vi "111_Setting.vi"() -> ()   [LabVIEW 2018]
panel:
  in  "偏移设定":T1
  in  "压销力":sgl[](array[numeric])
  in  "压销位移":sgl[](array[numeric])
  in  "内泄露":sgl[](array[numeric])
  in  "输入轴扭矩传感器":sgl[](array[numeric])
  in  "油压值":sgl[](array[numeric])
  # "传感器配置"
  # "量程下限"
  # "量程下限"
  # "量程下限"
  # "量程上限"
  # "量程上限"
  # "量程上限"
  # "量程下限"
  # "量程下限"
  # "量程上限"
  # "量程上限"
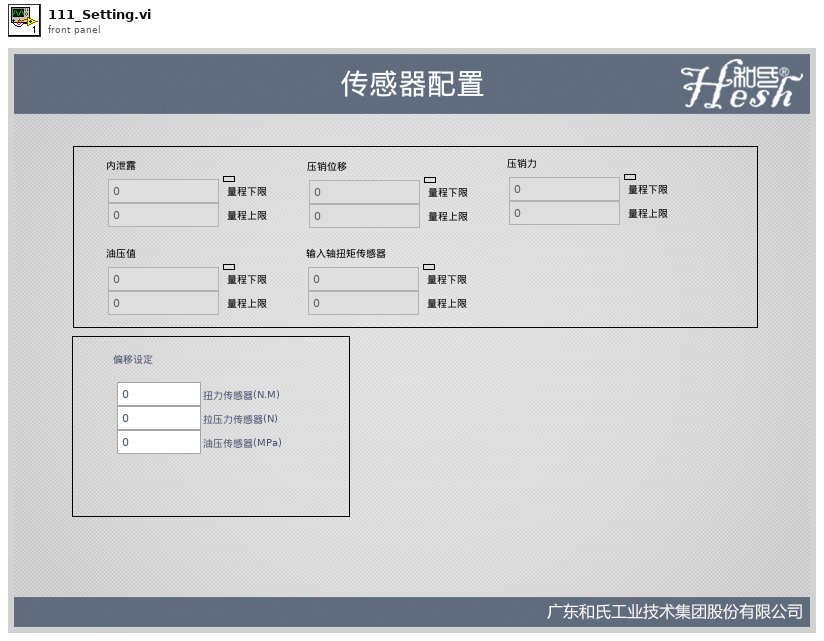
[diagram p1: front panel]
types:
  T1 = cluster{"扭力传感器(N.M)":dbl, "拉压力传感器(N)":dbl, "油压传感器(MPa) ":dbl}
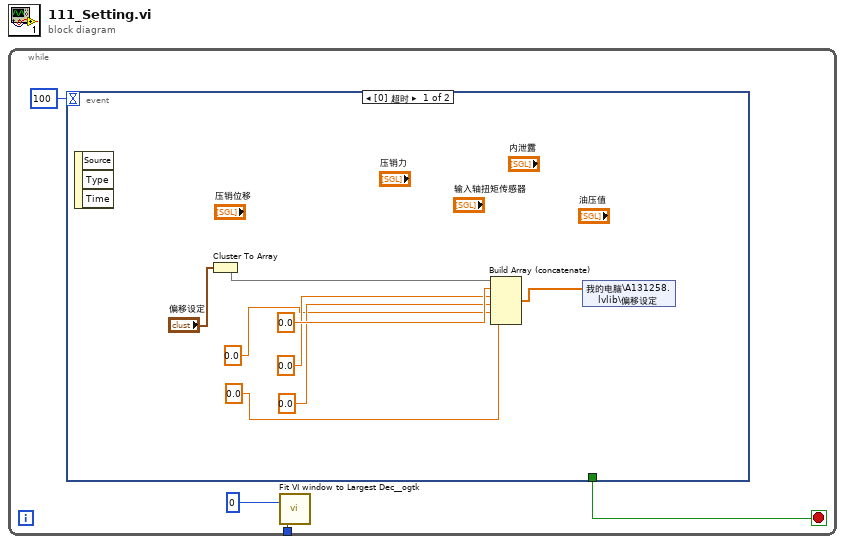
[diagram p0: block diagram]
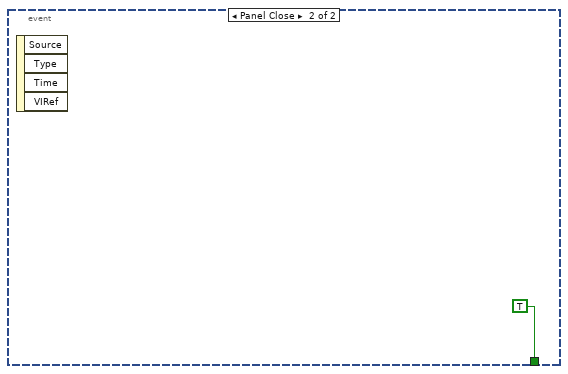
[diagram p2: hidden frame]
diagram:
  n1 = while {
    tunnel: [0 ("border spacing (2 px)")] -> w1
    stop <- w4 stop-if-true
    n2 = event shown="[0] 超时" {
      selector: _ -> [_ _]
      dyn-events: _ -> [_ _]
      timeout: 100 -> [_ _]
      tunnel: [_ TRUE] -> w4
      event Timeout {
        n3 = event-data() -> ()  [unwired: 1 in, 3 out]
        n4 = Cluster To Array(cluster="偏移设定") -> (array=w12:dbl[])
        n5 = Build Array (concatenate)(w12, sgl 0.0, sgl 0.0, sgl 0.0, sgl 0.0, sgl 0.0) -> (w11:dbl[])
        n6 = shared-variable "我的电脑\\A131258.lvlib\\偏移设定"(w11) -> ()  [unwired: 1 in, 1 out]
      }
      event Panel Close {
        n7 = event-data() -> ()  [unwired: 1 in, 4 out]
      }
    }
  }
  n8 = call <userlib>:"Fit VI window to Largest Dec__ogtk.vi"("border spacing (2 px)"=w1) -> ()  [unwired: 5 in, 2 out]
